vi "SplitString.vi"(10 "Separator":string, 11 "String[in]":string) -> (3 "Slices":string[](array[string]))   [LabVIEW 2013]
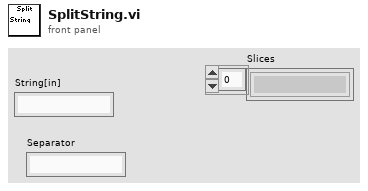
[diagram p1: front panel]
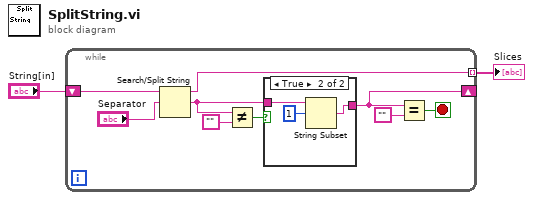
[diagram p0: block diagram]
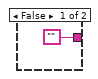
[diagram p2: hidden frame]
diagram:
  n1 = while {
    shift-right: [w3] -> _
    shift-left: "String[in]" -> [w10]
    tunnel: [w9] -> w1 mode=indexing
    stop <- w11 stop-if-true
    n2 = Search/Split String(string=w10, search string/char (-)="Separator") -> (substring before match=w9:string, match + rest of string=w7:string)  [unwired: 1 in, 1 out]
    n3 = Not Equal?(x=w7, y="") -> (x != y?=w8:bool)
    n4 = case shown="True" w8 {
      tunnel: w7 -> [_ w15]
      tunnel: ["" w13] -> w3
      frame False {
      }
      frame True {
        n5 = String Subset(string=w15, offset (0)=1) -> (substring=w13:string)  [unwired: 1 in]
      }
    }
    n6 = Equal?(x=w3, y="") -> (x = y?=w11:bool)
  }
  "Slices" <- w1
